vi "Actor Core.vi"(8 "error in":errorcluster, 11 "ActorMeter in":refnum<class "ActorMeter.lvclass">) -> (0 "error out":errorcluster, 3 "Actor out":refnum<class "Actor.lvclass">)   [LabVIEW 2014, in "ActorMeter.lvclass"]
doc: "(<B>Filename</B>: Actor Framework.lvlib:Actor.lvclass:Actor Core.vi)\n\nReceives messages to the actor, reacts to them, and initiates any error handling that may shut the actor down.\n\nDescendant classes may override this VI to append parallel tasks for the actor to complete while it handles messages. Overrides use the Call Parent Method node."
uses:
  ActorMeter.lvclass
  <vilib>/ActorFramework/Actor/Actor.lvclass
  ActorMeter.lvclass/ActorMeter.ctl
  <vilib>/ActorFramework/Actor/Actor.lvclass/Actor.ctl
  <vilib>/ActorFramework/Message Enqueuer/Message Enqueuer.lvclass/Message Enqueuer.ctl
  ActorMeter Messages/Show Child In Sub Panel Msg/Show Child In Sub Panel Msg.lvclass/Show Child In Sub Panel Msg.ctl
  <vilib>/ActorFramework/Message Enqueuer/Init from Existing Queue.vi
  <vilib>/ActorFramework/Message Enqueuer/Enqueue.vi
  <vilib>/ActorFramework/Message Priority Queue/Priority Enqueue.vi
  <vilib>/ActorFramework/Message Enqueuer/Message Enqueuer.lvclass
  <vilib>/ActorFramework/Stop Msg/Stop Msg.lvclass
  ActorMeter Messages/Show Child In Sub Panel Msg/Show Child In Sub Panel Msg.lvclass
  Interfaces/Observable Actor/Observable Actor.lvclass
panel:
  in  "Stop":bool
  in  "Tab Control":T1(tab)
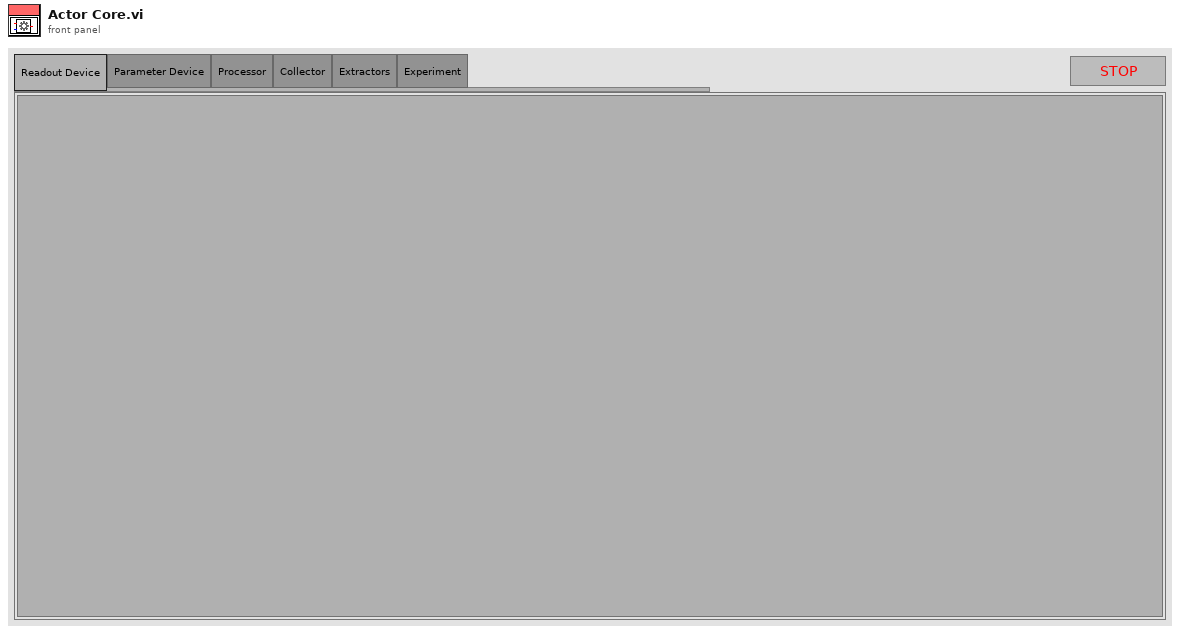
[diagram p1: front panel]
types:
  T1 = enum32{"Readout Device", "Parameter Device", "Processor", "Collector", "Extractors", "Experiment"}
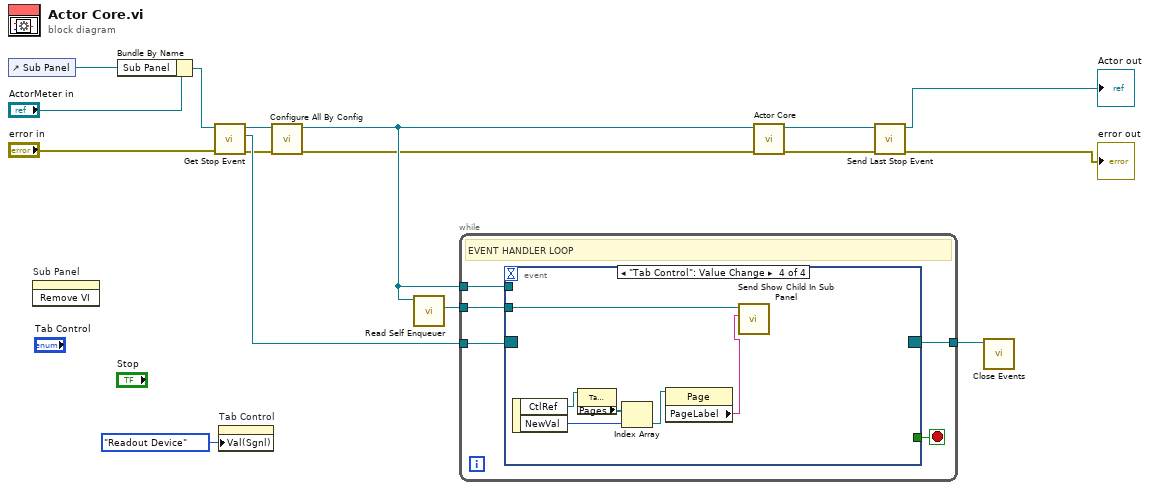
[diagram p0: block diagram]
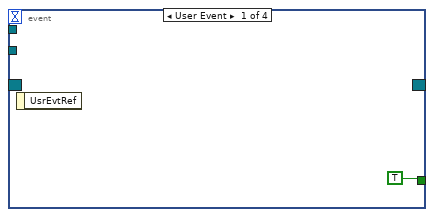
[diagram p2: hidden frame]
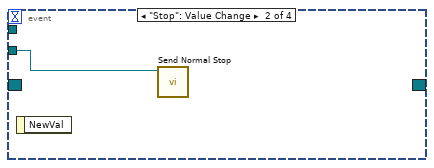
[diagram p3: hidden frame]
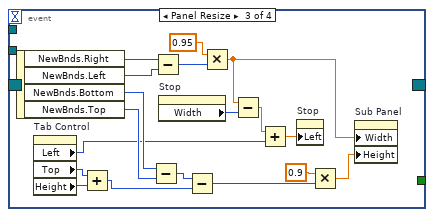
[diagram p4: hidden frame]
diagram:
  n1 = control-ref of="Sub Panel"() -> (w6:refnum<vi>)
  n2 = invoke on="Sub Panel" class="SubPanel" method="Remove VI"() -> ()  [unwired: 3 in, 3 out]
  n3 = Bundle By Name(cluster="ActorMeter in", "Sub Panel"=w6) -> (w7:refnum<class "ActorMeter.lvclass">)
  n4 = call-dynamic "Get Stop Event.vi"("error in (no error)"="error in", "Observable Actor in"=w7) -> ("error out"=w2:errorcluster, "Events"=w14:refnum<event-registration>, "Observable Actor out"=w3:refnum<class "ActorMeter.lvclass">)  [unwired: 7 in]
  n5 = property on="Tab Control" class="TabCtl (strict)"("Val(Sgnl)"=T1."Readout Device" ("Value (Signaling)")) -> ()  [unwired: 2 in, 2 out]
  n6 = call "Configure All By Config.vi"("error in"=w2, "ActorMeter in"=w3) -> ("error out"=w1:errorcluster, "ActorMeter out"=w4:refnum<class "ActorMeter.lvclass">)  [unwired: 8 in]
  n7 = call <vilib>:"Read Self Enqueuer.vi"("Actor"=w4) -> ("Self Enqueuer"=w16:refnum<class "Message Enqueuer.lvclass">)  [unwired: 10 in]
  n8 = while {
    tunnel: w14 -> [w21]
    tunnel: w16 -> [w20]
    tunnel: [w19] -> w11
    tunnel: w4 -> [w17]
    stop <- w18 stop-if-true
    # "EVENT HANDLER LOOP"
    n9 = event shown="[3] \"Tab Control\": Value Change" {
      selector: w21 -> [_ _ _ _]
      dyn-events: [_ _ _ _] -> w19
      timeout: _ -> [_ _ _ _]
      tunnel: w20 -> [_ w23 _ w42]
      tunnel: [TRUE _ _ _] -> w18
      tunnel: w17 -> [_ _ _ _]
      event User Event {
        n10 = event-data() -> ()  [unwired: 1 in, 1 out]
      }
      event "Stop": Value Change {
        n11 = event-data() -> ()  [unwired: 1 in, 1 out]
        n12 = call <vilib>:"Send Normal Stop.vi"("Message Enqueuer"=w23) -> ()  [unwired: 10 in, 1 out]
      }
      event Panel Resize {
        n13 = event-data() -> ("NewBnds.Right"=w34:i16, "NewBnds.Left"=w25:i16, "NewBnds.Bottom"=w33:i16, "NewBnds.Top"=w35:i16)  [unwired: 1 in]
        n14 = property on="Tab Control" class="TabCtl (strict)"() -> ("Left"=w24:i32, "Top"=w36:i32, "Height"=w37:u32)  [unwired: 2 in, 2 out]
        n15 = Add(x=w36, y=w37) -> (x+y=w31:u32)
        n16 = Subtract(x=w33, y=w35) -> (x-y=w32:i16)
        n17 = Subtract(x=w34, y=w25) -> (x-y=w41:i16)
        n18 = property on="Stop" class="Bool"() -> ("Width"=w28:u32)  [unwired: 2 in, 2 out]
        n19 = Subtract(x=w32, y=w31) -> (x-y=w30:u32)
        n20 = Multiply(x=0.95, y=w41) -> (x*y=w29:dbl)
        n21 = Subtract(x=w29, y=w28) -> (x-y=w26:dbl)
        n22 = Add(x=w26, y=w24) -> (x+y=w27:dbl)
        n23 = property on="Stop" class="Bool"("Left"=w27) -> ()  [unwired: 2 in, 2 out]
        n24 = Multiply(x=0.9, y=w30) -> (x*y=w38:dbl)
        n25 = property on="Sub Panel" class="SubPnl"("Width"=w29, "Height"=w38) -> ()  [unwired: 2 in, 2 out]
      }
      event "Tab Control": Value Change {
        n26 = event-data() -> ("CtlRef"=w47:refnum<vi>, "NewVal"=w44:T1)  [unwired: 1 in]
        n27 = property class="TabCtl (strict)"(reference=w47) -> ("Pages"=w46:refnum<vi>[])  [unwired: 1 in, 2 out]
        n28 = Index Array(array=w46, index=w44) -> (element=w45:refnum<vi>)
        n29 = property class="Page"(reference=w45) -> ("PageLabel"=w43:string)  [unwired: 1 in, 2 out]
        n30 = call "Send Show Child In Sub Panel.vi"("Child name"=w43, "Message Enqueuer"=w42) -> ()  [unwired: 8 in, 2 out]
      }
    }
  }
  n31 = call-parent "Actor Core.vi"("error in"=w1, "Actor in"=w4) -> ("error out"=w12:errorcluster, "Actor out"=w13:refnum<class "Actor.lvclass">)  [unwired: 8 in]
  n32 = call "Send Last Stop Event.vi"("error in (no error)"=w12, "Actor in"=w13) -> ("error out"=→"error out":errorcluster, "Actor  out"=→"Actor out":refnum<class "Actor.lvclass">)  [unwired: 8 in]
  n33 = call "Close Events.vi"("events"=w11) -> ()  [unwired: 11 in]
